vi "restore_config.vi"(3 "Auto Load Default?":bool) -> ()   [LabVIEW 2011]
doc: "Restores the chirp pulse experiment settings from a config file."
uses:
  <vilib>/Utility/config.llb/Read Key (I32).vi
  global.vi
  <vilib>/Utility/config.llb/Read Key (Boolean).vi
  <vilib>/Utility/config.llb/Read Key (Double).vi
  <vilib>/Utility/config.llb/Read Key (String).vi
  <vilib>/Utility/config.llb/Read Key (Path).vi
  <vilib>/Utility/config.llb/NI_LVConfig.lvlib
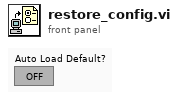
[diagram p1: front panel]
types:
  T1 = typedef "NI_LVConfig.lvlib/Config Data RefNum.ctl" = refnum<k1>
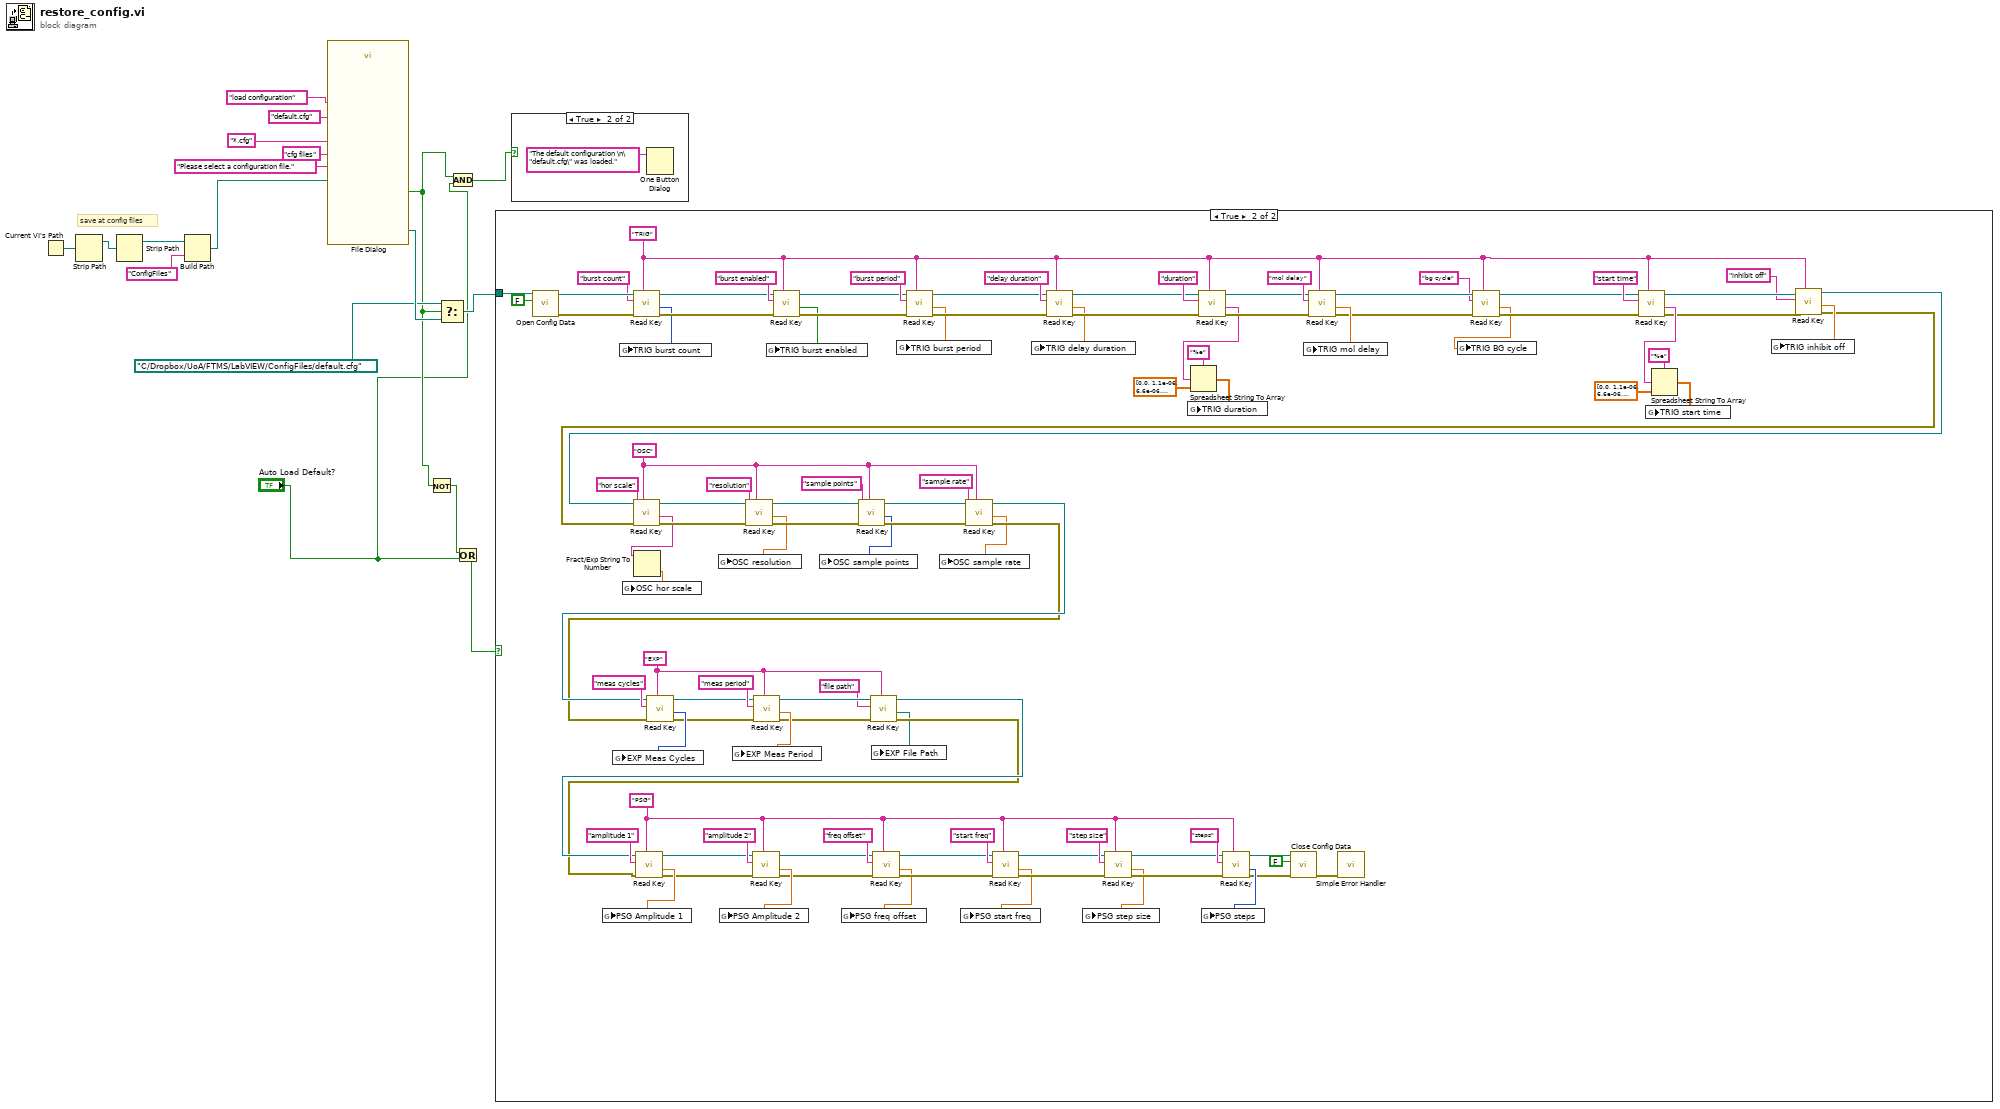
[diagram p0: block diagram]
diagram:
  # "save at config files"
  n1 = Current VI's Path() -> (path=w13:path)
  n2 = Strip Path(path=w13) -> (stripped path=w11:path)  [unwired: 1 out]
  n3 = Strip Path(path=w11) -> (stripped path=w10:path)  [unwired: 1 out]
  n4 = Build Path(base path=w10, name or relative path="ConfigFiles") -> (appended path=w9:path)
  n5 = call "File Dialog"("start path"=w9, "prompt"="Please select a configuration file.", "button label"="load configuration", "default name"="default.cfg", "pattern (all files)"="*.cfg" ("default name"), "pattern label"="cfg files") -> ("selected path"=w8:path, "cancelled"=w2:bool)  [unwired: 6 in, 2 out]
  n6 = Not(x=w2) -> (.not. x?=w4:bool)
  n7 = Select(t=path "C:/Dropbox/UoA/FTMS/LabVIEW/ConfigFiles/default.cfg", s=w2, f=w8) -> (s? t:f=w6:path)
  n8 = And(x=w2, y="Auto Load Default?") -> (x .and. y?=w3:bool)
  n9 = Or(x=w4, y="Auto Load Default?") -> (x .or. y?=w5:bool)
  n10 = case shown="True" w5 {
    tunnel: w6 -> [_ w123]
    frame False {
    }
    frame True {
      w51 = "PSG"
      w21 = "EXP"
      w92 = "OSC"
      w26 = "TRIG"
      n11 = call <vilib>:"Open Config Data.vi"("create file if necessary (T)"=FALSE, "configuration file path"=w123) -> ("error out"=w121:errorcluster, "refnum"=w122:T1)  [unwired: 1 in, 7 out]
      n12 = call-poly <vilib>:"Read Key.vi"("section"=w26, "error in (no error)"=w121, "key"="burst count" ("Key 1"), "refnum"=w122) -> ("error out"=w110:errorcluster, "value"=w77:i32, "refnum out"=w114:T1)  [unwired: 4 in, 1 out]
      n13 = global write "global.vi" "TRIG burst count"(w77) -> ()
      n14 = call-poly <vilib>:"Read Key.vi"("section"=w26, "error in (no error)"=w110, "key"="burst enabled" ("Key 1"), "refnum"=w114) -> ("error out"=w109:errorcluster, "value"=w76:bool, "refnum out"=w113:T1)  [unwired: 4 in, 1 out]
      n15 = global write "global.vi" "TRIG burst enabled"(w76) -> ()
      n16 = call-poly <vilib>:"Read Key.vi"("section"=w26, "error in (no error)"=w109, "key"="burst period" ("Key 1"), "refnum"=w113) -> ("error out"=w108:errorcluster, "value"=w75:dbl, "refnum out"=w112:T1)  [unwired: 4 in, 1 out]
      n17 = global write "global.vi" "TRIG burst period"(w75) -> ()
      n18 = call-poly <vilib>:"Read Key.vi"("section"=w26, "error in (no error)"=w108, "key"="delay duration" ("Key 1"), "refnum"=w112) -> ("error out"=w107:errorcluster, "value"=w74:dbl, "refnum out"=w111:T1)  [unwired: 4 in, 1 out]
      n19 = global write "global.vi" "TRIG delay duration"(w74) -> ()
      n20 = call-poly <vilib>:"Read Key.vi"("section"=w26, "error in (no error)"=w107, "key"="duration" ("Key 1"), "refnum"=w111) -> ("error out"=w103:errorcluster, "value"=w71:string, "refnum out"=w104:T1)  [unwired: 4 in, 1 out]
      n21 = Spreadsheet String To Array(format string="%e", spreadsheet string=w71, array type (2D Dbl)=dbl[] [0.0, 1.1e-06, 6.6e-06, 6.4e-06] ("TRIG start time")) -> (array=w72:dbl[])  [unwired: 1 in]
      n22 = global write "global.vi" "TRIG duration"(w72) -> ()
      n23 = call-poly <vilib>:"Read Key.vi"("section"=w26, "error in (no error)"=w103, "key"="mol delay" ("Key 1"), "refnum"=w104) -> ("error out"=w36:errorcluster, "value"=w66:dbl, "refnum out"=w35:T1)  [unwired: 4 in, 1 out]
      n24 = global write "global.vi" "TRIG mol delay"(w66) -> ()
      n25 = call-poly <vilib>:"Read Key.vi"("section"=w26, "error in (no error)"=w36, "key"="bg cycle" ("Key 1"), "refnum"=w35) -> ("error out"=w37:errorcluster, "value"=w33:dbl, "refnum out"=w38:T1)  [unwired: 4 in, 1 out]
      n26 = global write "global.vi" "TRIG BG cycle"(w33) -> ()
      n27 = call-poly <vilib>:"Read Key.vi"("section"=w26, "error in (no error)"=w37, "key"="start time" ("Key 1"), "refnum"=w38) -> ("error out"=w31:errorcluster, "value"=w65:string, "refnum out"=w32:T1)  [unwired: 4 in, 1 out]
      n28 = Spreadsheet String To Array(format string="%e", spreadsheet string=w65, array type (2D Dbl)=dbl[] [0.0, 1.1e-06, 6.6e-06, 6.4e-06] ("TRIG start time")) -> (array=w68:dbl[])  [unwired: 1 in]
      n29 = global write "global.vi" "TRIG start time"(w68) -> ()
      n30 = call-poly <vilib>:"Read Key.vi"("section"=w26, "error in (no error)"=w31, "key"="inhibit off" ("Key 1"), "refnum"=w32) -> ("error out"=w27:errorcluster, "value"=w29:dbl, "refnum out"=w28:T1)  [unwired: 4 in, 1 out]
      n31 = call-poly <vilib>:"Read Key.vi"("section"=w92, "error in (no error)"=w27, "key"="hor scale" ("Key 1"), "refnum"=w28) -> ("error out"=w97:errorcluster, "value"=w44:string, "refnum out"=w99:T1)  [unwired: 4 in, 1 out]
      n32 = Fract/Exp String To Number(string=w44) -> (number=w43:dbl)  [unwired: 3 in, 1 out]
      n33 = global write "global.vi" "OSC hor scale"(w43) -> ()
      n34 = call-poly <vilib>:"Read Key.vi"("section"=w92, "error in (no error)"=w97, "key"="resolution" ("Key 1"), "refnum"=w99) -> ("error out"=w96:errorcluster, "value"=w64:dbl, "refnum out"=w98:T1)  [unwired: 4 in, 1 out]
      n35 = global write "global.vi" "OSC resolution"(w64) -> ()
      n36 = call-poly <vilib>:"Read Key.vi"("section"=w92, "error in (no error)"=w96, "key"="sample points" ("Key 1"), "refnum"=w98) -> ("error out"=w93:errorcluster, "value"=w63:i32, "refnum out"=w94:T1)  [unwired: 4 in, 1 out]
      n37 = global write "global.vi" "OSC sample points"(w63) -> ()
      n38 = call-poly <vilib>:"Read Key.vi"("section"=w92, "error in (no error)"=w93, "key"="sample rate" ("Key 1"), "refnum"=w94) -> ("error out"=w89:errorcluster, "value"=w62:dbl, "refnum out"=w90:T1)  [unwired: 4 in, 1 out]
      n39 = call-poly <vilib>:"Read Key.vi"("section"=w21, "error in (no error)"=w89, "key"="meas cycles" ("Key 1"), "refnum"=w90) -> ("error out"=w40:errorcluster, "value"=w61:i32, "refnum out"=w41:T1)  [unwired: 4 in, 1 out]
      n40 = global write "global.vi" "EXP Meas Cycles"(w61) -> ()
      n41 = call-poly <vilib>:"Read Key.vi"("section"=w21, "error in (no error)"=w40, "key"="meas period" ("Key 1"), "refnum"=w41) -> ("error out"=w24:errorcluster, "value"=w39:dbl, "refnum out"=w25:T1)  [unwired: 4 in, 1 out]
      n42 = global write "global.vi" "EXP Meas Period"(w39) -> ()
      n43 = call-poly <vilib>:"Read Key.vi"("section"=w21, "error in (no error)"=w24, "key"="file path", "refnum"=w25) -> ("error out"=w22:errorcluster, "value"=w19:path, "refnum out"=w23:T1)  [unwired: 4 in, 1 out]
      n44 = call-poly <vilib>:"Read Key.vi"("section"=w51, "error in (no error)"=w22, "key"="amplitude 1" ("Key 1"), "refnum"=w23) -> ("error out"=w46:errorcluster, "value"=w54:dbl, "refnum out"=w48:T1)  [unwired: 4 in, 1 out]
      n45 = global write "global.vi" "PSG Amplitude 1"(w54) -> ()
      n46 = call-poly <vilib>:"Read Key.vi"("section"=w51, "error in (no error)"=w46, "key"="amplitude 2" ("Key 1"), "refnum"=w48) -> ("error out"=w45:errorcluster, "value"=w52:dbl, "refnum out"=w47:T1)  [unwired: 4 in, 1 out]
      n47 = global write "global.vi" "PSG Amplitude 2"(w52) -> ()
      n48 = global write "global.vi" "EXP File Path"(w19) -> ()
      n49 = call-poly <vilib>:"Read Key.vi"("section"=w51, "error in (no error)"=w45, "key"="freq offset" ("Key 1"), "refnum"=w47) -> ("error out"=w83:errorcluster, "value"=w60:dbl, "refnum out"=w85:T1)  [unwired: 4 in, 1 out]
      n50 = global write "global.vi" "PSG freq offset"(w60) -> ()
      n51 = global write "global.vi" "OSC sample rate"(w62) -> ()
      n52 = call-poly <vilib>:"Read Key.vi"("section"=w51, "error in (no error)"=w83, "key"="start freq" ("Key 1"), "refnum"=w85) -> ("error out"=w82:errorcluster, "value"=w59:dbl, "refnum out"=w84:T1)  [unwired: 4 in, 1 out]
      n53 = global write "global.vi" "PSG start freq"(w59) -> ()
      n54 = call-poly <vilib>:"Read Key.vi"("section"=w51, "error in (no error)"=w82, "key"="step size" ("Key 1"), "refnum"=w84) -> ("error out"=w79:errorcluster, "value"=w58:dbl, "refnum out"=w80:T1)  [unwired: 4 in, 1 out]
      n55 = global write "global.vi" "PSG step size"(w58) -> ()
      n56 = call-poly <vilib>:"Read Key.vi"("section"=w51, "error in (no error)"=w79, "key"="steps" ("Key 1"), "refnum"=w80) -> ("error out"=w49:errorcluster, "value"=w57:i32, "refnum out"=w50:T1)  [unwired: 4 in, 1 out]
      n57 = global write "global.vi" "PSG steps"(w57) -> ()
      n58 = call <vilib>:"Close Config Data.vi"("error in (no error)"=w49, "write file if changed (T)"=FALSE, "refnum"=w50) -> ("error out"=w119:errorcluster)  [unwired: 8 out]
      n59 = call <vilib>:"Simple Error Handler.vi"("error in (no error)"=w119) -> ()  [unwired: 1 in, 8 out]
      n60 = global write "global.vi" "TRIG inhibit off"(w29) -> ()
    }
  }
  n61 = case shown="True" w3 {
    frame False {
    }
    frame True {
      n62 = One Button Dialog(message="The default configuration \n\"default.cfg\" was loaded.") -> ()  [unwired: 1 in, 1 out]
    }
  }
